vi "带启用输入端的反馈节点.vi"() -> ()   [LabVIEW 2020]
panel:
  out "result":dbl
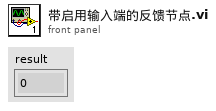
[diagram p1: front panel]
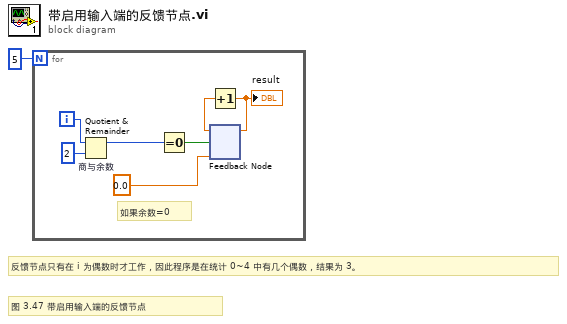
[diagram p0: block diagram]
diagram:
  # "图 3.47 带启用输入端的反馈节点"
  # "反馈节点只有在 i 为偶数时才工作，因此程序是在统计 0~4 中有几个偶数，结果为 3。"
  n1 = for {
    N: 5 -> [_]
    i -> [w3]
    # "如果余数=0"
    n2 = Quotient & Remainder "商与余数"(x=w3, y=2) -> (x-y*floor(x/y)=w4:i32)  [unwired: 1 out]
    n3 = Equal To 0?(x=w4) -> (x = 0?=w2:bool)
    n4 = feedback #1(0.0) -> (w7:dbl)
    n5 = Increment(x=w7) -> (x+1=w8:dbl)
    "result" <- w8
    n6 = feedback-in #1(w8, w2) -> ()
  }
